vi "2526 Connect.vi"(8 "error in (no error)":errorcluster, 9 "Index":i32, 10 "2525 Scan List Channels":string[](array[string]), 11 "IVI Refnum in":refnum<k15>) -> (0 "error out":errorcluster, 3 "IVI Refnum out":refnum<k15>)   [LabVIEW 2019, in "SupportVIs.lvlib"]
uses:
  SupportVIs.lvlib
  <instrlib>/niSwitch/niSwitch.llb/niSwitch Connect Channels (Single).vi
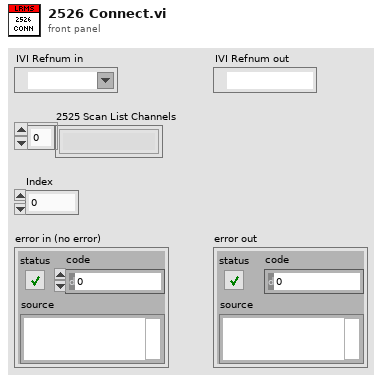
[diagram p1: front panel]
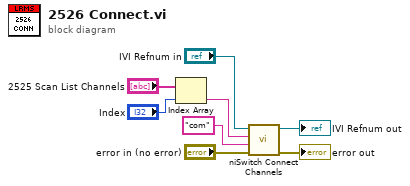
[diagram p0: block diagram]
diagram:
  n1 = Index Array(array="2525 Scan List Channels", index="Index") -> (element=w2:string)
  n2 = call-poly <instrlib>:"niSwitch Connect Channels.vi"("error in (no error)"="error in (no error)", "channel 2"="com", "channel 1"=w2, "instrument handle"="IVI Refnum in") -> ("error out"=→"error out":errorcluster, "instrument handle out"=→"IVI Refnum out":refnum<k15>)  [unwired: 6 in]
